vi "SysDef.Property.Get.vi"   [LabVIEW 2027, in "Advanced System Definition.lvlib"]
uses:
  Advanced System Definition.lvlib
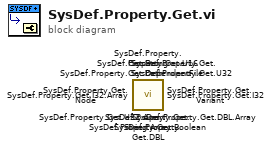
[diagram p0: block diagram]
diagram:
  n1 = call "SysDef.Property.Get.String.Array.vi"() -> ()  [unwired: 8 in, 4 out]
  n2 = call "SysDef.Property.Get.DependentFile.vi"() -> ()  [unwired: 8 in, 4 out]
  n3 = call "SysDef.Property.Get.Node.vi"() -> ()  [unwired: 8 in, 4 out]
  n4 = call "SysDef.Property.Get.Variant.vi"() -> ()  [unwired: 8 in, 4 out]
  n5 = call "SysDef.Property.Get.Path.vi"() -> ()  [unwired: 8 in, 4 out]
  n6 = call "SysDef.Property.Get.String.vi"() -> ()  [unwired: 8 in, 4 out]
  n7 = call "SysDef.Property.Get.DBL.Array.vi"() -> ()  [unwired: 8 in, 4 out]
  n8 = call "SysDef.Property.Get.DBL.vi"() -> ()  [unwired: 8 in, 4 out]
  n9 = call <vilib>:"SysDef.Property.Get.I32.Array.vi"() -> ()  [unwired: 8 in, 4 out]
  n10 = call "SysDef.Property.Get.I32.vi"() -> ()  [unwired: 8 in, 4 out]
  n11 = call "SysDef.Property.Get.U32.Array.vi"() -> ()  [unwired: 8 in, 4 out]
  n12 = call <vilib>:"SysDef.Property.Get.U32.vi"() -> ()  [unwired: 8 in, 4 out]
  n13 = call <vilib>:"SysDef.Property.Get.U16.vi"() -> ()  [unwired: 8 in, 4 out]
  n14 = call <vilib>:"SysDef.Property.Get.Boolean.vi"() -> ()  [unwired: 8 in, 4 out]
